vi "Table Stage Front Panel Settings.vi"(7 "Actions":T1=enum."Defer FP Update", 8 "Error In":errorcluster, 11 "This VI":refnum<vi>) -> (0 "Error Out":errorcluster)   [LabVIEW 2014]
uses:
  Controls/Table Stage GUI Front Panel Configurator AFGV Actions.ctl
  <vilib>/Utility/miscctls.llb/LVPointTypeDef.ctl
  <vilib>/Utility/miscctls.llb/LVRectTypeDef.ctl
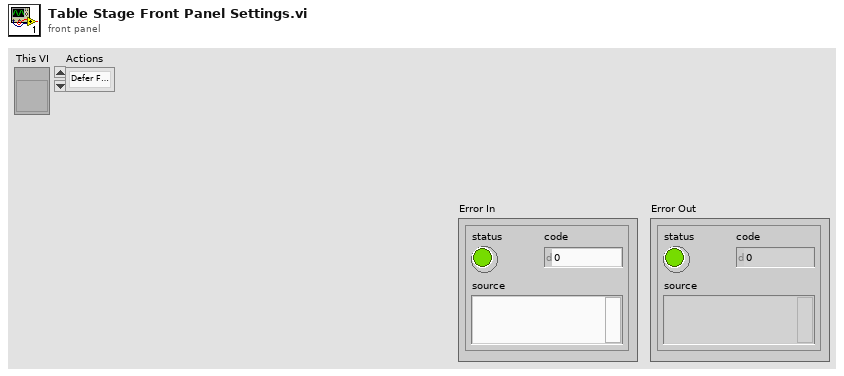
[diagram p1: front panel]
types:
  T1 = typedef "Table Stage GUI Front Panel Configurator AFGV Actions.ctl" = enum16{"Init", "Defer FP Update", "Enable FP Update", "Disable Ctrls", "Enable Ctrls", "Basic", "Advanced"}
  T2 = typedef "LVPointTypeDef.ctl" = cluster{"Horizontal":i16, "Vertical":i16}
  T3 = typedef "LVRectTypeDef.ctl" = cluster{"Left":i16, "Top":i16, "Right":i16, "Bottom":i16}
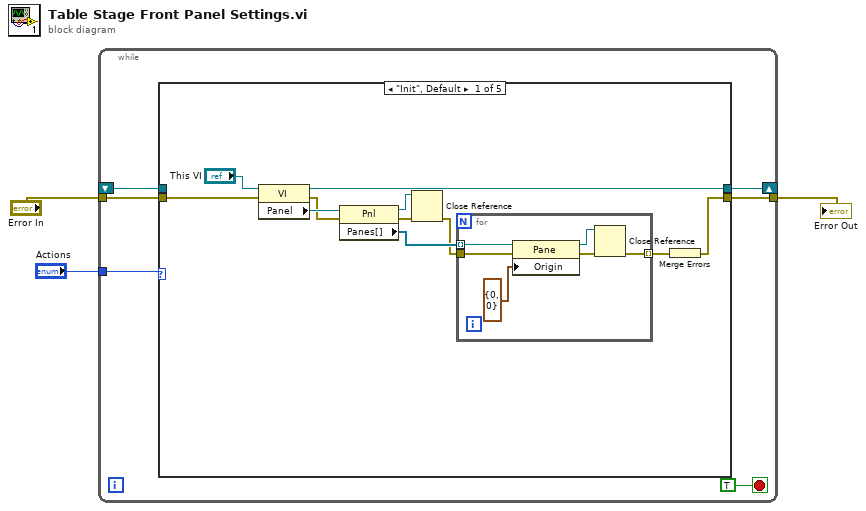
[diagram p0: block diagram]
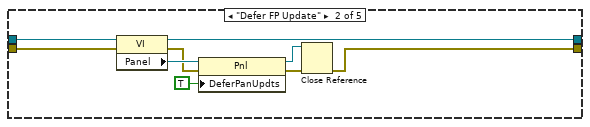
[diagram p2: hidden frame]
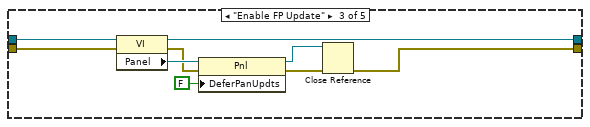
[diagram p3: hidden frame]
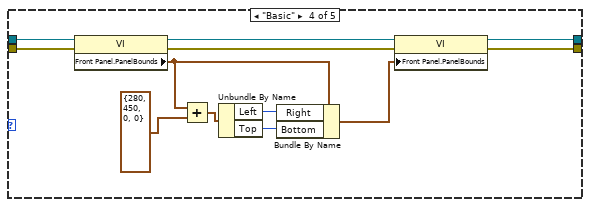
[diagram p4: hidden frame]
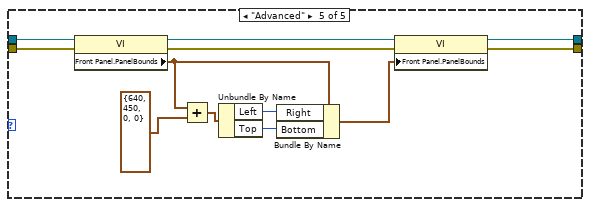
[diagram p5: hidden frame]
diagram:
  n1 = while {
    tunnel: "Actions" -> [w9]
    shift-right: [w7] -> _
    shift-left: _ -> [w6]
    tunnel: [w5] -> w2
    tunnel: "Error In" -> [w4]
    stop <- TRUE stop-if-true
    n2 = case shown="\"Init\", Default" w9 {
      tunnel: [w18 w33 w42 w50 w62] -> w7
      tunnel: w6 -> [_ w34 w43 w56 w68]
      tunnel: [w10 w27 w37 w52 w64] -> w5
      tunnel: w4 -> [w20 w35 w44 w54 w66]
      frame "Init", Default {
        n3 = property class="VI"(reference="This VI", error in=w20) -> (reference out=w18:refnum<vi>, error out=w15:errorcluster, "Panel"=w17:refnum<vi>)
        n4 = property class="Pnl"(reference=w17, error in=w15) -> (reference out=w13:refnum<vi>, error out=w14:errorcluster, "Panes[]"=w16:refnum<vi>[])
        n5 = Close Reference(reference=w13, error in (no error)=w14) -> (error out=w12:errorcluster)
        n6 = for {
          tunnel: w16 -> [w26] mode=indexing
          tunnel: w12 -> [w24]
          tunnel: [w21] -> w11 mode=indexing
          n7 = property class="Pane"(reference=w26, error in=w24, "Origin"=T2 {"Horizontal"=0, "Vertical"=0}) -> (reference out=w22:refnum<vi>, error out=w23:errorcluster)
          n8 = Close Reference(reference=w22, error in (no error)=w23) -> (error out=w21:errorcluster)
        }
        n9 = Merge Errors(w11) -> (w10:errorcluster)
      }
      frame "Defer FP Update" {
        n10 = property class="VI"(reference=w34, error in=w35) -> (reference out=w33:refnum<vi>, error out=w31:errorcluster, "Panel"=w32:refnum<vi>)
        n11 = property class="Pnl"(reference=w32, error in=w31, "DeferPanUpdts"=TRUE ("Defer Panel Updates")) -> (reference out=w28:refnum<vi>, error out=w29:errorcluster)
        n12 = Close Reference(reference=w28, error in (no error)=w29) -> (error out=w27:errorcluster)
      }
      frame "Enable FP Update" {
        n13 = property class="VI"(reference=w43, error in=w44) -> (reference out=w42:refnum<vi>, error out=w40:errorcluster, "Panel"=w41:refnum<vi>)
        n14 = property class="Pnl"(reference=w41, error in=w40, "DeferPanUpdts"=FALSE ("Defer Panel Updates")) -> (reference out=w36:refnum<vi>, error out=w39:errorcluster)
        n15 = Close Reference(reference=w36, error in (no error)=w39) -> (error out=w37:errorcluster)
      }
      frame "Basic" {
        n16 = property class="VI"(reference=w56, error in=w54) -> (reference out=w51:refnum<vi>, error out=w55:errorcluster, "Front Panel.PanelBounds"=w49:T3)
        n17 = Add(x=w49, y=T3 {"Left"=280, "Top"=450, "Right"=0, "Bottom"=0} ("Front Panel Window:Panel Bounds")) -> (x+y=w48:T3)
        n18 = Unbundle By Name(w48) -> ("Left"=w47:i16, "Top"=w46:i16)
        n19 = Bundle By Name(cluster=w49, "Right"=w47, "Bottom"=w46) -> (w45:T3)
        n20 = property class="VI"(reference=w51, error in=w55, "Front Panel.PanelBounds"=w45) -> (reference out=w50:refnum<vi>, error out=w52:errorcluster)
      }
      frame "Advanced" {
        n21 = property class="VI"(reference=w68, error in=w66) -> (reference out=w63:refnum<vi>, error out=w67:errorcluster, "Front Panel.PanelBounds"=w61:T3)
        n22 = Add(x=w61, y=T3 {"Left"=640, "Top"=450, "Right"=0, "Bottom"=0} ("Front Panel Window:Panel Bounds")) -> (x+y=w60:T3)
        n23 = Unbundle By Name(w60) -> ("Left"=w59:i16, "Top"=w58:i16)
        n24 = Bundle By Name(cluster=w61, "Right"=w59, "Bottom"=w58) -> (w57:T3)
        n25 = property class="VI"(reference=w63, error in=w67, "Front Panel.PanelBounds"=w57) -> (reference out=w62:refnum<vi>, error out=w64:errorcluster)
      }
    }
  }
  "Error Out" <- w2
